vi "pipe.vi"() -> ()   [LabVIEW 2017]
uses:
  Pedestal LW/Labview/DLL/PipeDLL.dll
panel:
  out "STS":i32
  in  "arg2":dbl
  in  "arg1":dbl
  in  "stop":bool
  out "SetPipe":i32
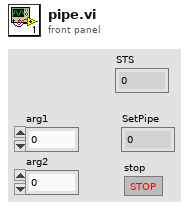
[diagram p1: front panel]
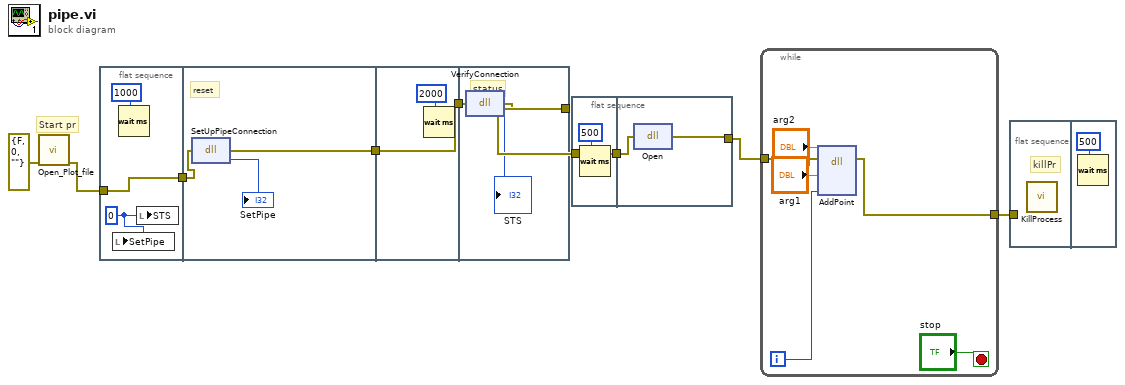
[diagram p0: block diagram]
diagram:
  # "Start pr"
  n1 = call "Open_Plot_file.vi"("error in"=errorcluster {"status"=FALSE, "code"=0, "source"=""}) -> ("error out"=w8:errorcluster)  [unwired: 7 in, 3 out]
  n2 = flat-sequence {
    tunnel: [w11] -> w7
    tunnel: w8 -> [w11]
    tunnel: w7 -> [w14]
    tunnel: [w13] -> w6
    tunnel: w6 -> [w16]
    tunnel: [w16] -> w5
    tunnel: w5 -> [w20]
    tunnel: [w19] -> w4
    frame #0 {
      w10 = 0 ("STS")
      n3 = local write "SetPipe"(w10) -> ()
      n4 = Wait (ms)(milliseconds to wait=u32 1000) -> ()  [unwired: 1 out]
      n5 = local write "STS"(w10) -> ()
    }
    frame #1 {
      # "reset"
      n6 = dll-call lib="C:/Projects/Pedestal LW/Labview/DLL/PipeDLL.dll" fn="SetUpPipeConnection"(error in=w14) -> (error out=w13:errorcluster, "return type"=→"SetPipe":i32)  [unwired: 2 in, 1 out]
    }
    frame #2 {
      n7 = Wait (ms)(milliseconds to wait=u32 2000) -> ()  [unwired: 1 out]
    }
    frame #3 {
      # "status"
      n8 = dll-call lib="C:/Projects/Pedestal LW/Labview/DLL/PipeDLL.dll" fn="VerifyConnection"(error in=w20) -> (error out=w19:errorcluster, "return type"=→"STS":i32)  [unwired: 2 in, 1 out]
    }
  }
  n9 = flat-sequence {
    tunnel: w4 -> [w21]
    tunnel: [w21] -> w3
    tunnel: w3 -> [w24]
    tunnel: [w23] -> w2
    frame #0 {
      n10 = Wait (ms)(milliseconds to wait=u32 500) -> ()  [unwired: 1 out]
    }
    frame #1 {
      n11 = dll-call lib="C:/Projects/Pedestal LW/Labview/DLL/PipeDLL.dll" fn="Open"(error in=w24) -> (error out=w23:errorcluster)  [unwired: 3 in, 1 out]
    }
  }
  n12 = while {
    tunnel: w2 -> [w29]
    tunnel: [w28] -> w1
    i -> [w25]
    stop <- "stop" stop-if-true
    n13 = dll-call lib="C:/Projects/Pedestal LW/Labview/DLL/PipeDLL.dll" fn="AddPoint"(error in=w29, "arg1"="arg1", "arg2"="arg2", "time"=w25) -> (error out=w28:errorcluster)  [unwired: 6 in, 1 out]
  }
  n14 = flat-sequence {
    tunnel: w1 -> [_]
    frame #0 {
      # "killPr"
      n15 = call "KillProcess.vi"() -> ()  [unwired: 12 in]
    }
    frame #1 {
      n16 = Wait (ms)(milliseconds to wait=u32 500) -> ()  [unwired: 1 out]
    }
  }
